vi "Build CHM.vi"() -> ()   [LabVIEW 2020]
uses:
  <vilib>/Utility/config.llb/Read Key (String).vi
  <vilib>/Utility/config.llb/Read Key (Path).vi
  <vilib>/NI/Compiled HTML Menu Tool/CHM Generator/CHM Generator.lvclass
  <vilib>/Utility/config.llb/NI_LVConfig.lvlib
panel:
  out "error out":errorcluster
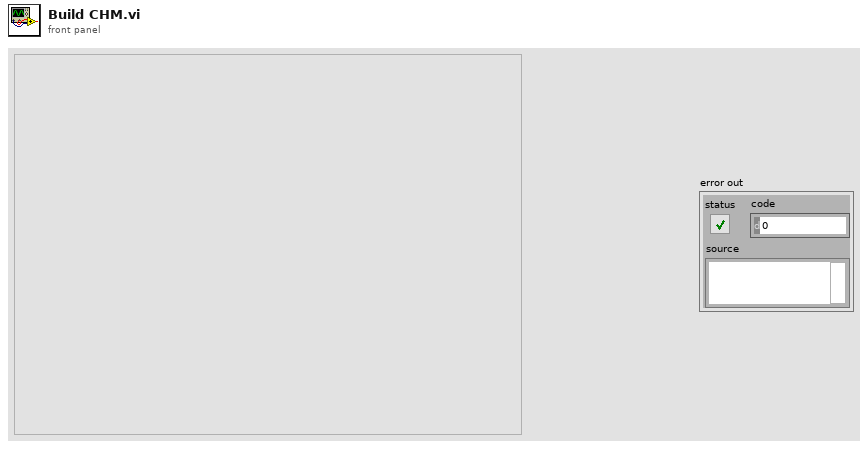
[diagram p1: front panel]
types:
  T1 = typedef "NI_LVConfig.lvlib/Config Data RefNum.ctl" = refnum<k1>
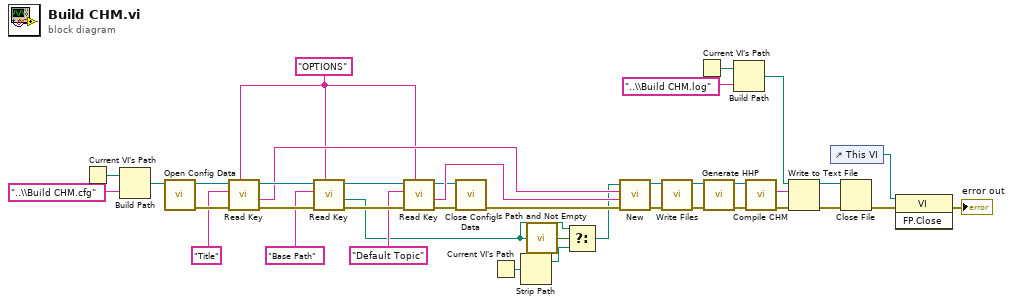
[diagram p0: block diagram]
diagram:
  w20 = "OPTIONS" ("section")
  n1 = Current VI's Path() -> (path=w19:path)
  n2 = Build Path(base path=w19, name or relative path="..\\Build CHM.cfg") -> (appended path=w17:path)
  n3 = call <vilib>:"Open Config Data.vi"("configuration file path"=w17) -> ("error out"=w32:errorcluster, "refnum"=w33:T1)  [unwired: 8 in, 1 out]
  n4 = call-poly <vilib>:"Read Key.vi"("section"=w20, "error in (no error)"=w32, "key"="Title", "refnum"=w33) -> ("error out"=w30:errorcluster, "value"=w27:string, "refnum out"=w29:T1)  [unwired: 4 in, 1 out]
  n5 = call-poly <vilib>:"Read Key.vi"("section"=w20, "error in (no error)"=w30, "key"="Base Path", "refnum"=w29) -> ("error out"=w26:errorcluster, "value"=w3:path, "refnum out"=w25:T1)  [unwired: 4 in, 1 out]
  n6 = call-poly <vilib>:"Read Key.vi"("section"=w20, "error in (no error)"=w26, "key"="Default Topic", "refnum"=w25) -> ("error out"=w22:errorcluster, "value"=w23:string, "refnum out"=w21:T1)  [unwired: 4 in, 1 out]
  n7 = call <vilib>:"Close Config Data.vi"("error in (no error)"=w22, "refnum"=w21) -> ("error out"=w7:errorcluster)  [unwired: 8 in, 1 out]
  n8 = Current VI's Path() -> (path=w5:path)
  n9 = Strip Path(path=w5) -> (stripped path=w4:path)  [unwired: 1 out]
  n10 = call <vilib>:"Is Path and Not Empty.vi"("path"=w3) -> ("Is Path and Not Empty?"=w6:bool)  [unwired: 4 in]
  n11 = Select(t=w3, s=w6, f=w4) -> (s? t:f=w2:path)
  n12 = call <vilib>:"New.vi"("error in (no error)"=w7, "Default topic"=w23, "Title"=w27, "Base Path"=w2) -> ("error out"=w38:errorcluster, "CHM Generator out"=w39:refnum<class "CHM Generator.lvclass">)  [unwired: 6 in]
  n13 = call-dynamic "Write Files.vi"("error in (no error)"=w38, "CHM Generator in"=w39) -> ("error out"=w37:errorcluster, "CHM Generator out"=w36:refnum<class "CHM Generator.lvclass">)  [unwired: 8 in]
  n14 = Current VI's Path() -> (path=w16:path)
  n15 = call-dynamic "Generate HHP.vi"("error in (no error)"=w37, "CHM Generator in"=w36) -> ("error out"=w34:errorcluster, "CHM Generator out"=w35:refnum<class "CHM Generator.lvclass">)  [unwired: 8 in]
  n16 = Build Path(base path=w16, name or relative path="..\\Build CHM.log") -> (appended path=w14:path)
  n17 = call <vilib>:"Compile CHM.vi"("error in (no error)"=w34, "CHM Generator in"=w35) -> ("error out"=w10:errorcluster, "standard output"=w13:string)  [unwired: 7 in, 1 out]
  n18 = Write to Text File(file (use dialog)=w14, text=w13, error in=w10) -> (refnum out=w11:refnum<file>, error out=w12:errorcluster)  [unwired: 1 in, 1 out]
  n19 = control-ref of="This VI"() -> (w9:refnum<vi>)
  n20 = Close File(refnum=w11, error in=w12) -> (error out=w8:errorcluster)  [unwired: 1 out]
  n21 = invoke class="VI" method="FP.Close"(reference=w9, error in=w8) -> (error out=→"error out":errorcluster)  [unwired: 1 in, 2 out]
